vi "Flywheel_Hardware_Begin.vi"(8 "error in":errorcluster) -> (0 "error out":errorcluster)   [LabVIEW 2020]
uses:
  <vilib>/Rock Robotics/WPI/ThirdParty/Phoenix-LabVIEW/Motor Controller/Controls/CTRE_Phoenix_MotorControl_SupplyCurrentLimitConfiguration.ctl
  <vilib>/Rock Robotics/WPI/ThirdParty/Phoenix-LabVIEW/Motor Controller/Controls/CTRE_Phoenix_MotorControl_TalonFXInvertType.ctl
  <vilib>/Rock Robotics/WPI/ThirdParty/Phoenix-LabVIEW/Motor Controller/Controls/CTRE_Phoenix_MotorControl_NeutralMode.ctl
  Flywheel_Hardware_Globals.vi
panel:
  in  "F":dbl=0.05
  in  "D":dbl=0.01
  in  "I":dbl
  in  "P":dbl=0.15
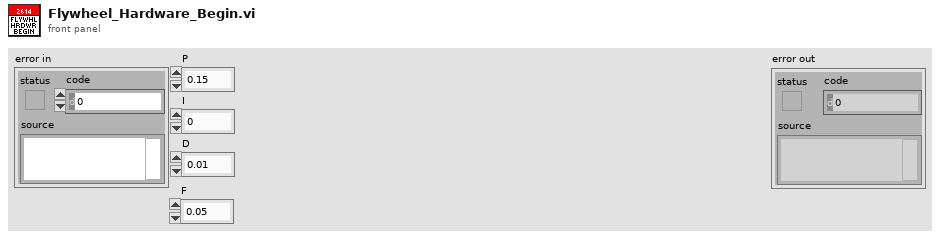
[diagram p1: front panel]
types:
  T1 = enum16{"FollowerType_PercentOutput", "FollowerType_AuxOutput1"}
  T2 = typedef "CTRE_Phoenix_MotorControl_NeutralMode.ctl" = enum8{"EEPROMSetting", "Override to Coast", "Override to Brake"}
  T3 = typedef "CTRE_Phoenix_MotorControl_TalonFXInvertType.ctl" = enum16{"Counter-Clockwise", "Clockwise"}
  T4 = typedef "CTRE_Phoenix_MotorControl_SupplyCurrentLimitConfiguration.ctl" = cluster{"Enable?":bool, "Current Limit":dbl, "Threshold Current":dbl, "Threshold Time":dbl}
  T5 = typedef "WPI_MotorControlDeviceRef.ctl" = cluster{"DeviceStatus":errorcluster, "Type":T6, "PWM":cluster{"PWM Channel":T7, "DeadBand":T8}, "CAN":cluster{"Device Number":u8, "SetOutput VI Ref":variant, "GetOutput VI Ref":variant, "Enable VI Ref":variant, "Disable VI Ref":variant, "Data":variant}, "Invert":bool, "DIO PWM":cluster{"PWM \"Enable\" Channel":T7, "DIOChannel":T9, "PWM Rate":dbl}}
  T6 = typedef "WPI_MotorControlType.ctl" = enum16{"PWM", "CAN", "DIO PWM"}
  T7 = typedef "FPGA_DIOPWMChannel.ctl" = enum8{"PWM 0", "PWM 1", "PWM 2", "PWM 3", "PWM 4", "PWM 5", "PWM 6", "PWM 7", "PWM 8", "PWM 9", "PWM MXP 0", "PWM MXP 1", "PWM MXP 2", "PWM MXP 3", "PWM MXP 4", "PWM MXP 5", "PWM MXP 6", "PWM MXP 7", "PWM MXP 8", "PWM MXP 9", "Invalid"}
  T8 = typedef "WPI_PWMDeadband.ctl" = cluster{"Name":string, "maxPositivePwm":i32, "minPositivePwm":i32, "centerPwm":i32, "maxNegativePwm":i32, "minNegativePwm":i32, "angularRange":u16}
  T9 = typedef "FPGA_DIOChannel.ctl" = enum8{"DIO 0", "DIO 1", "DIO 2", "DIO 3", "DIO 4", "DIO 5", "DIO 6", "DIO 7", "DIO 8", "DIO 9", "DIO MXP 0", "DIO MXP 1", "DIO MXP 2", "DIO MXP 3", "DIO MXP 4", "DIO MXP 5", "DIO MXP 6", "DIO MXP 7", "DIO MXP 8", "DIO MXP 9", "DIO MXP 10", "DIO MXP 11", "DIO MXP 12", "DIO MXP 13", "DIO MXP 14", "DIO MXP 15", "SPI Port CS1", "SPI Port CS2", "SPI Port CS3", "SPI Port MISO", "SPI Port MOSI", "Invalid"}
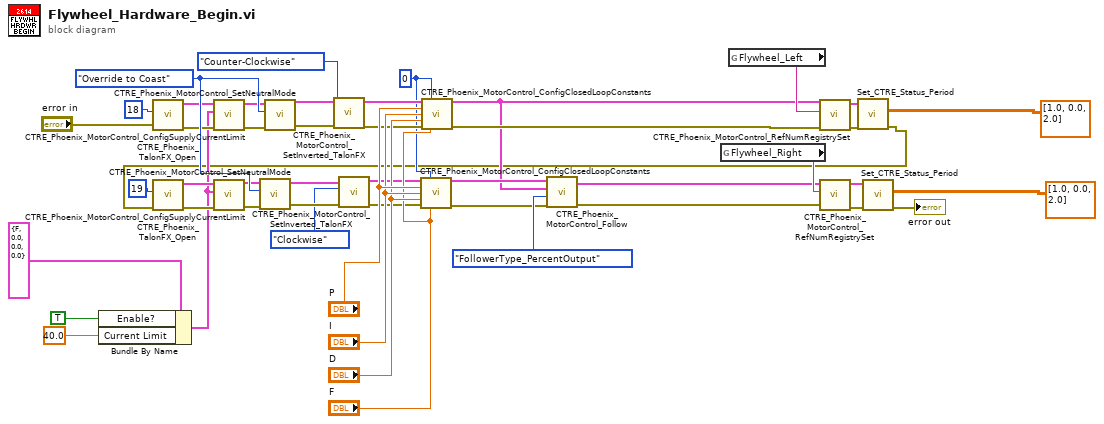
[diagram p0: block diagram]
diagram:
  w40 = CTRE_Phoenix_MotorControl_NeutralMode."Override to Coast" ("Motor Control Neutral Mode")
  w15 = 0 ("slotIdx")
  n1 = Bundle By Name(cluster=T4 {"Enable?"=FALSE, "Current Limit"=0.0, "Threshold Current"=0.0, "Threshold Time"=0.0} ("Supply Current Limit Configuration"), "Enable?"=TRUE, "Current Limit"=40.0) -> (w16:T4)
  n2 = call <vilib>:"CTRE_Phoenix_TalonFX_Open.vi"("error in"="error in", "Device Number"=u8 18) -> ("error out"=w26:errorcluster, "PhoenixMotorControlDevRef"=w27:T5)  [unwired: 8 in]
  n3 = call <vilib>:"CTRE_Phoenix_MotorControl_ConfigSupplyCurrentLimit.vi"("error in (no error)"=w26, "Supply Current Limit Configuration"=w16, "PhoenixMotorControlDevRef"=w27) -> ("error out"=w23:errorcluster, "PhoenixMotorControlDevRef"=w24:T5)  [unwired: 7 in]
  n4 = call <vilib>:"CTRE_Phoenix_MotorControl_SetNeutralMode.vi"("error in (no error)"=w23, "Motor Control Neutral Mode"=w40, "PhoenixMotorControlDevRef"=w24) -> ("error out"=w22:errorcluster, "PhoenixMotorControlDevRef"=w21:T5)  [unwired: 7 in]
  n5 = call <vilib>:"CTRE_Phoenix_MotorControl_SetInverted_TalonFX.vi"("error in (no error)"=w22, "Invert Type"=CTRE_Phoenix_MotorControl_TalonFXInvertType."Counter-Clockwise", "PhoenixMotorControlDevRef"=w21) -> ("error out"=w18:errorcluster, "PhoenixMotorControlDevRef"=w19:T5)  [unwired: 7 in]
  n6 = call <vilib>:"CTRE_Phoenix_MotorControl_ConfigClosedLoopConstants.vi"("PhoenixMotorControlDevRef"=w19, "slotIdx"=w15, "P"="P", "I"="I", "D"="D", "error in (no error)"=w18, "F"="F") -> ("PhoenixMotorControlDevRef"=w12:T5, "error out"=w17:errorcluster)  [unwired: 7 in]
  n7 = global read "Flywheel_Hardware_Globals.vi" "Flywheel_Right"() -> (w36:string)
  n8 = global read "Flywheel_Hardware_Globals.vi" "Flywheel_Left"() -> (w25:string)
  n9 = call <vilib>:"CTRE_Phoenix_MotorControl_RefNumRegistrySet.vi"("error in (no error)"=w17, "refnum name"=w25, "PhoenixMotorControlDevRef"=w12) -> ("error out"=w6:errorcluster, "PhoenixMotorControlDevRef"=w7:T5)  [unwired: 7 in]
  n10 = call "Set_CTRE_Status_Period.vi"("error in (no error)"=w6, "Frame Settings"=dbl[][] [[1.0], [0.0], [2.0]], "PhoenixMotorControlDevRef"=w7) -> ("error out"=w5:errorcluster)  [unwired: 7 in, 1 out]
  n11 = call <vilib>:"CTRE_Phoenix_TalonFX_Open.vi"("error in"=w5, "Device Number"=u8 19) -> ("error out"=w37:errorcluster, "PhoenixMotorControlDevRef"=w38:T5)  [unwired: 8 in]
  n12 = call <vilib>:"CTRE_Phoenix_MotorControl_ConfigSupplyCurrentLimit.vi"("error in (no error)"=w37, "Supply Current Limit Configuration"=w16, "PhoenixMotorControlDevRef"=w38) -> ("error out"=w34:errorcluster, "PhoenixMotorControlDevRef"=w35:T5)  [unwired: 7 in]
  n13 = call <vilib>:"CTRE_Phoenix_MotorControl_SetNeutralMode.vi"("error in (no error)"=w34, "Motor Control Neutral Mode"=w40, "PhoenixMotorControlDevRef"=w35) -> ("error out"=w32:errorcluster, "PhoenixMotorControlDevRef"=w33:T5)  [unwired: 7 in]
  n14 = call <vilib>:"CTRE_Phoenix_MotorControl_SetInverted_TalonFX.vi"("error in (no error)"=w32, "Invert Type"=CTRE_Phoenix_MotorControl_TalonFXInvertType."Clockwise", "PhoenixMotorControlDevRef"=w33) -> ("error out"=w29:errorcluster, "PhoenixMotorControlDevRef"=w30:T5)  [unwired: 7 in]
  n15 = call <vilib>:"CTRE_Phoenix_MotorControl_ConfigClosedLoopConstants.vi"("PhoenixMotorControlDevRef"=w30, "slotIdx"=w15, "P"="P", "I"="I", "D"="D", "error in (no error)"=w29, "F"="F") -> ("PhoenixMotorControlDevRef"=w13:T5, "error out"=w11:errorcluster)  [unwired: 7 in]
  n16 = call <vilib>:"CTRE_Phoenix_MotorControl_Follow.vi"("error in (no error)"=w11, "FollowerType"=T1."FollowerType_PercentOutput", "Master Controller to Follow"=w12, "PhoenixMotorControlDevRef"=w13) -> ("error out"=w9:errorcluster, "PhoenixMotorControlDevRef"=w10:T5)  [unwired: 6 in]
  n17 = call <vilib>:"CTRE_Phoenix_MotorControl_RefNumRegistrySet.vi"("error in (no error)"=w9, "refnum name"=w36, "PhoenixMotorControlDevRef"=w10) -> ("error out"=w2:errorcluster, "PhoenixMotorControlDevRef"=w3:T5)  [unwired: 7 in]
  n18 = call "Set_CTRE_Status_Period.vi"("error in (no error)"=w2, "Frame Settings"=dbl[][] [[1.0], [0.0], [2.0]], "PhoenixMotorControlDevRef"=w3) -> ("error out"=→"error out":errorcluster)  [unwired: 7 in, 1 out]
